vi "Lookup APIs of Type.vi"(8 "error in (no error)":errorcluster, 9 "Futures:Promise":refnum<class "Promise.lvclass">, 10 "Identity - Type Only":refnum<class "Identity.lvclass">, 11 "VolatusCore in":refnum<class "VolatusCore.lvclass">) -> (0 "error out":errorcluster, 3 "VolatusCore out":refnum<class "VolatusCore.lvclass">)   [LabVIEW 2020, in "Volatus.lvlib" / "VolatusCore.lvclass"]
uses:
  VolatusCore.lvclass
  Identity/Identity.lvclass
  VolatusCore.lvclass/VolatusCore.ctl
  ApiArrayValue/ApiArrayValue.lvclass
  lv-promises/Promises/Promise/Promise.lvclass
  C:/dev/lv20CE/relink/lv-promises/Promises/Value/Value.lvclass
  C:/dev/lv20CE/relink/lv-volatus/Volatus/ApiArrayValue/ApiArrayValue.lvclass
  API/API.lvclass
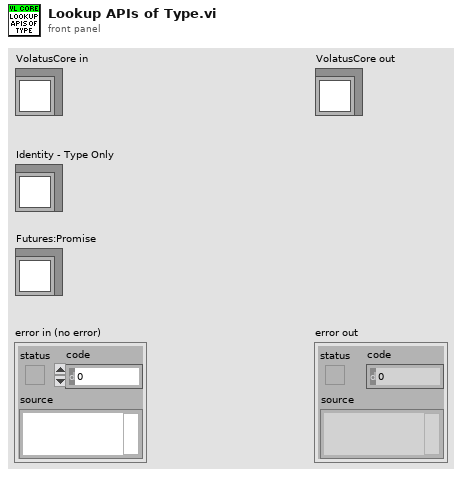
[diagram p1: front panel]
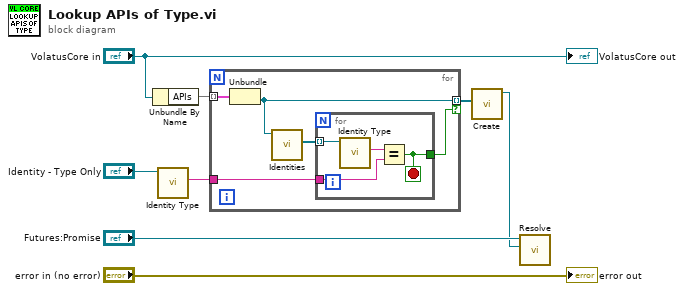
[diagram p0: block diagram]
diagram:
  n1 = Unbundle By Name("VolatusCore in") -> ("APIs"=w4:map{u32, refnum<class "API.lvclass">})
  n2 = call-dynamic "Identity Type.vi"("Identity in"="Identity - Type Only") -> ("Type"=w5:string)  [unwired: 10 in]
  n3 = for {
    tunnel: w5 -> [w11]
    tunnel: w4 -> [w13] mode=indexing
    tunnel: [w10] -> w3 mode=indexing if=w9
    n4 = Unbundle(w13) -> ("API"=w10:refnum<class "API.lvclass">)  [unwired: 1 out]
    n5 = call-dynamic "Identities.vi"("API in"=w10) -> ("Identities"=w12:refnum<class "Identity.lvclass">[])  [unwired: 8 in, 2 out]
    n6 = for {
      tunnel: w12 -> [w17] mode=indexing
      tunnel: w11 -> [w15]
      tunnel: [w14] -> w9
      stop <- w14 stop-if-true
      n7 = call-dynamic "Identity Type.vi"("Identity in"=w17) -> ("Type"=w16:string)  [unwired: 10 in]
      n8 = Equal?(x=w16, y=w15) -> (x = y?=w14:bool)
    }
  }
  n9 = call "Create.vi"("APIs"=w3) -> ("ApiArrayValue out"=w1:refnum<class "ApiArrayValue.lvclass">)  [unwired: 10 in]
  n10 = call "Resolve.vi"("Result"=w1, "Promise in"="Futures:Promise") -> ()  [unwired: 8 in, 2 out]
  "error out" <- "error in (no error)"
  "VolatusCore out" <- "VolatusCore in"
